vi "Get File Name.vi"(8 "error in":errorcluster, 11 "reference in":refnum<class "Electronic Datasheet.lvclass">) -> (0 "error out":errorcluster, 2 "File Name":string, 3 "reference out":refnum<class "Electronic Datasheet.lvclass">)   [LabVIEW 2020, in "Electronic Datasheet.lvlib" / "Electronic Datasheet.lvclass"]
uses:
  Electronic Datasheet.lvclass
  Electronic Datasheet.lvclass/Electronic Datasheet.ctl
  Core/File Info/File Info.lvclass
  <vilib>/Utility/Data Type/NI_Data Type.lvlib
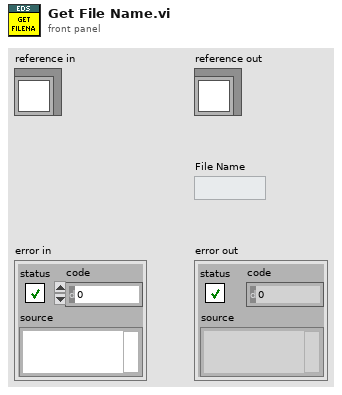
[diagram p1: front panel]
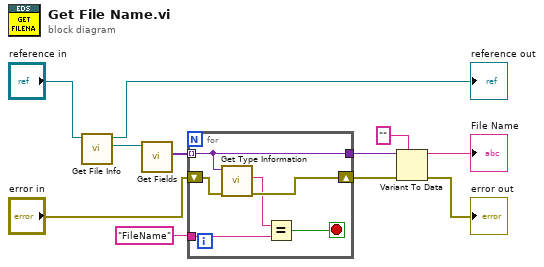
[diagram p0: block diagram]
diagram:
  n1 = call "Get File Info.vi"("reference in"="reference in") -> ("File Info"=w9:refnum<class "File Info.lvclass">, "reference out"=→"reference out":refnum<class "Electronic Datasheet.lvclass">)  [unwired: 9 in]
  n2 = call-dynamic "Get Fields.vi"("File Info in"=w9) -> ("Fields"=w1:variant[])  [unwired: 9 in, 1 out]
  n3 = for {
    tunnel: w1 -> [w17] mode=indexing
    tunnel: [w17] -> w4
    shift-right: [w16] -> w3
    shift-left: "error in" -> [w15]
    tunnel: "FileName" ("element") -> [w13]
    stop <- w14 stop-if-true
    n4 = call <vilib>:"Get Type Information.vi"("error in (no error)"=w15, "variant"=w17) -> ("error out"=w16:errorcluster, "name"=w12:string)  [unwired: 5 in, 3 out]
    n5 = Equal?(x=w12, y=w13) -> (x = y?=w14:bool)
  }
  n6 = Variant To Data(error in=w3, type="", Variant=w4) -> (data=→"File Name":string, error out=→"error out":errorcluster)
